vi "Update Slot Configuration.vi"(6 "Max # of Racks":u32, 8 "error in (no error)":errorcluster, 9 "Card Position":T1[](array[typedef]) {"Slot #" max=15}, 10 "Card Name":string[](array[string]), 11 "Slot Configuration in":refnum<vi>) -> (0 "error out":errorcluster, 3 "Slot Configuration out":refnum<vi>)   [LabVIEW 2014, in "SLSC configuration System Explorer.lvlib"]
uses:
  SLSC configuration System Explorer.lvlib
  Type Defs/Card Position.ctl
  Shared/SPI Utility/Slot #.ctl
  <vilib>/Utility/miscctls.llb/LVRowAndColumnTypeDef.ctl
  Shared/Constants.vi
  Shared/SLSC configuration Shared.lvlib
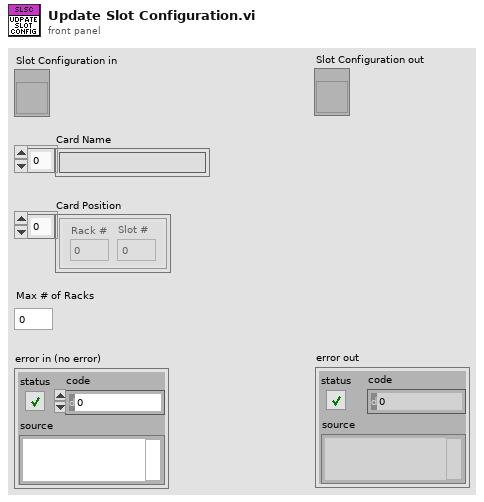
[diagram p1: front panel]
types:
  T1 = typedef "SLSC configuration Shared.lvlib/Card Position.ctl" = cluster{"Rack #":u8, "Slot #":T2}
  T2 = typedef "SLSC configuration Shared.lvlib/Slot #.ctl" = u8
  T3 = typedef "LVRowAndColumnTypeDef.ctl" = cluster{"Row":i32, "Column":i32}
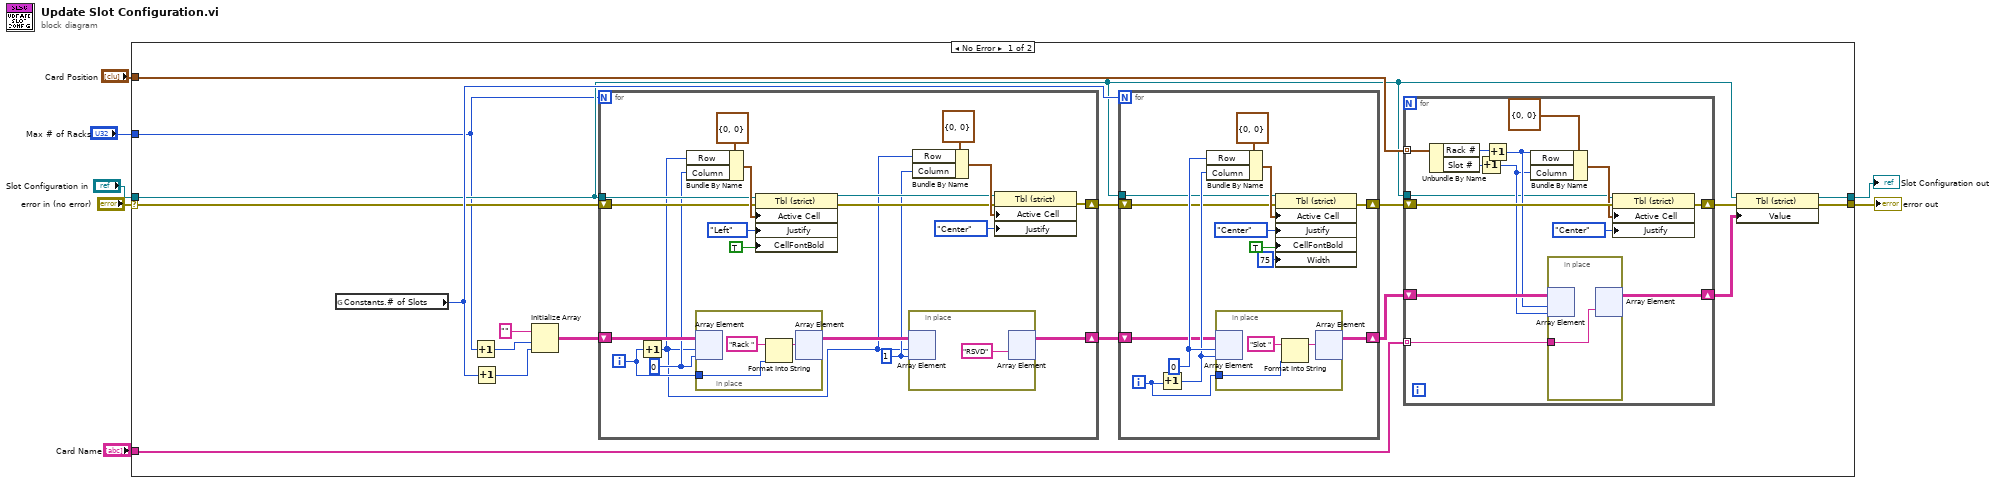
[diagram p0: block diagram]
diagram:
  n1 = case shown="No Error" "error in (no error)" {
    selector: "error in (no error)" -> [w14 w80]
    tunnel: "Card Position" -> [w23 _]
    tunnel: "Card Name" -> [w22 _]
    tunnel: [w12 w80] -> w2
    tunnel: "Slot Configuration in" -> [w9 w81]
    tunnel: [w10 w81] -> w3
    tunnel: "Max # of Racks" -> [w8 _]
    frame No Error {
      n2 = global read "Constants.vi" "Constants.# of Slots"() -> (w15:u8)
      n3 = Increment(x=w8) -> (x+1=w24:u32)
      n4 = Increment(x=w15) -> (x+1=w16:u8)
      n5 = Initialize Array("", w24, w16) -> (w21:string[][])
      n6 = for {
        N: w8 -> [_]
        shift-right: [w43] -> w20
        shift-left: w21 -> [w60]
        shift-right: [w46] -> w19
        shift-left: w14 -> [w56]
        tunnel: w9 -> [w55]
        i -> [w45]
        w44 = 1
        w53 = 0
        n7 = Increment(x=w45) -> (x+1=w42:i32)
        n8 = Bundle By Name(cluster=T3 {"Row"=0, "Column"=0} ("Active Cell:Active Cell"), "Row"=w42, "Column"=w53) -> (w58:T3)
        n9 = in-place {
          in-place-border: w45 -> [w64]
          n10 = in-place-array #1(w60, w42, w53) -> ()  [unwired: 1 out]
          n11 = Format Into String(initial string="Rack ", w64) -> (resulting string=w62:string)  [unwired: 2 in, 1 out]
          n12 = in-place-array #1(w62) -> (w52:string[][])  [unwired: 2 out]
        }
        n13 = property class="Tbl (strict)"(reference=w55, error in=w56, "Active Cell"=w58, "Justify"=enum16{"Left", "Center", "Right"}."Left" ("Active Cell:Cell Justification"), "CellFontBold"=TRUE ("Active Cell:Cell Font:Bold")) -> (reference out=w47:refnum<vi>, error out=w48:errorcluster)
        n14 = in-place {
          n15 = in-place-array #2(w52, w42, w44) -> ()  [unwired: 1 out]
          n16 = in-place-array #2("RSVD" ("initial string")) -> (w43:string[][])  [unwired: 2 out]
        }
        n17 = Bundle By Name(cluster=T3 {"Row"=0, "Column"=0} ("Active Cell:Active Cell"), "Row"=w42, "Column"=w44) -> (w50:T3)
        n18 = property class="Tbl (strict)"(reference=w47, error in=w48, "Active Cell"=w50, "Justify"=enum16{"Left", "Center", "Right"}."Center" ("Active Cell:Cell Justification")) -> (error out=w46:errorcluster)  [unwired: 1 out]
      }
      n19 = for {
        N: w15 -> [_]
        shift-right: [w28] -> w18
        shift-left: w20 -> [w29]
        shift-right: [w27] -> w17
        shift-left: w19 -> [w31]
        tunnel: w9 -> [w30]
        i -> [w34]
        w33 = 0
        n20 = Increment(x=w34) -> (x+1=w32:i32)
        n21 = Bundle By Name(cluster=T3 {"Row"=0, "Column"=0} ("Active Cell:Active Cell"), "Row"=w33, "Column"=w32) -> (w37:T3)
        n22 = in-place {
          in-place-border: w34 -> [w41]
          n23 = in-place-array #3(w29, w33, w32) -> ()  [unwired: 1 out]
          n24 = Format Into String(initial string="Slot ", w41) -> (resulting string=w39:string)  [unwired: 2 in, 1 out]
          n25 = in-place-array #3(w39) -> (w28:string[][])  [unwired: 2 out]
        }
        n26 = property class="Tbl (strict)"(reference=w30, error in=w31, "Active Cell"=w37, "Justify"=enum16{"Left", "Center", "Right"}."Center" ("Active Cell:Cell Justification"), "CellFontBold"=TRUE ("Active Cell:Cell Font:Bold"), "Width"=u32 75 ("Active Cell:Cell Size:Width")) -> (error out=w27:errorcluster)  [unwired: 1 out]
      }
      n27 = for {
        tunnel: w23 -> [w77] mode=indexing
        shift-right: [w70] -> w11
        shift-left: w18 -> [w72]
        tunnel: w22 -> [w71] mode=indexing
        shift-right: [w73] -> w13
        shift-left: w17 -> [w78]
        tunnel: w9 -> [w65]
        n28 = Unbundle By Name(w77) -> ("Rack #"=w68:u8, "Slot #"=w69:T2)
        n29 = Increment(x=w69) -> (x+1=w66:T2)
        n30 = Increment(x=w68) -> (x+1=w67:u8)
        n31 = Bundle By Name(cluster=T3 {"Row"=0, "Column"=0} ("Active Cell:Active Cell"), "Row"=w67, "Column"=w66) -> (w75:T3)
        n32 = in-place {
          in-place-border: w71 -> [w79]
          n33 = in-place-array #4(w72, w67, w66) -> ()  [unwired: 1 out]
          n34 = in-place-array #4(w79) -> (w70:string[][])  [unwired: 2 out]
        }
        n35 = property class="Tbl (strict)"(reference=w65, error in=w78, "Active Cell"=w75, "Justify"=enum16{"Left", "Center", "Right"}."Center" ("Active Cell:Cell Justification")) -> (error out=w73:errorcluster)  [unwired: 1 out]
      }
      n36 = property class="Tbl (strict)"(reference=w9, error in=w13, "Value"=w11) -> (reference out=w10:refnum<vi>, error out=w12:errorcluster)
    }
    frame Error {
    }
  }
  "error out" <- w2
  "Slot Configuration out" <- w3
